vi "Is Connected.vi"(8 "error in (no error)":errorcluster, 9 "Raise error if not connected":bool, 11 "WAMP Client in":refnum<class "WAMP Client.lvclass">) -> (0 "error out":errorcluster, 1 "Is Connected?":bool, 3 "WAMP Client out":refnum<class "WAMP Client.lvclass">)   [LabVIEW 2020, in "wamplv.lvlib" / "WAMP Client.lvclass"]
uses:
  WAMP Client.lvclass
  WAMP Client.lvclass/WAMP Client.ctl
  <vilib>/Utility/error.llb/Error Cluster From Error Code.vi
  <vilib>/ErrorRing/Error Ring.xnode
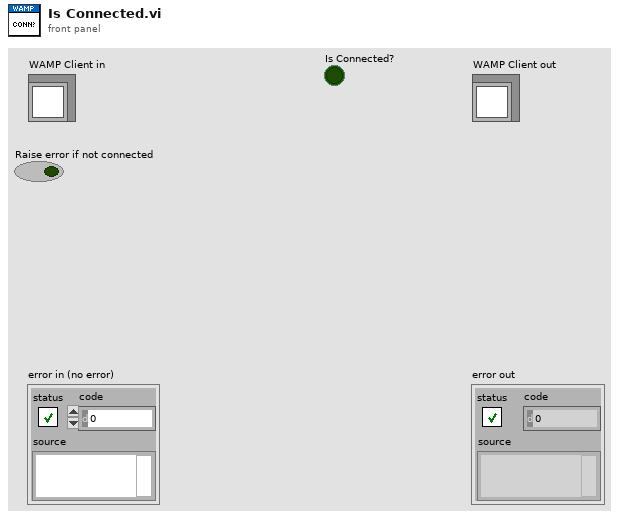
[diagram p1: front panel]
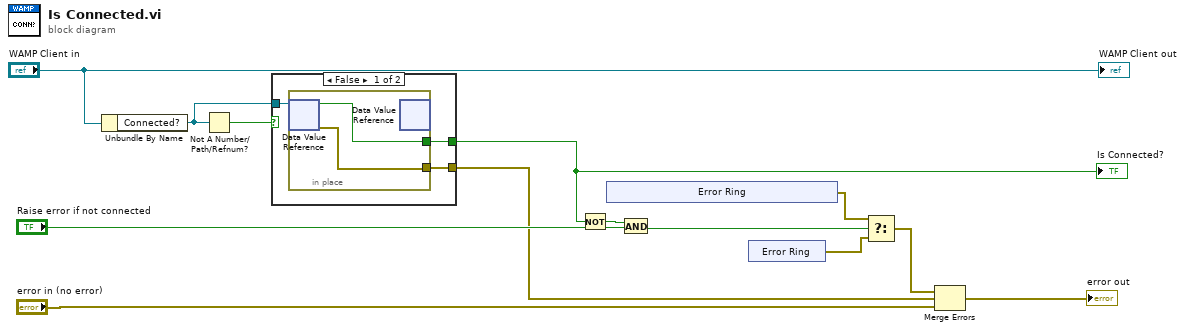
[diagram p0: block diagram]
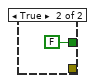
[diagram p2: hidden frame]
diagram:
  n1 = Unbundle By Name("WAMP Client in") -> ("Connected?"=w1:refnum<data-value>)
  n2 = Not A Number/Path/Refnum?(number/path/refnum=w1) -> (NaN/Path/Refnum?=w2:bool)
  n3 = case shown="False" w2 {
    tunnel: [w16 FALSE] -> w12
    tunnel: [w15 _] -> w5
    tunnel: w1 -> [w14 _]
    frame False {
      n4 = in-place {
        in-place-border: [w18] -> w16
        in-place-border: [w17] -> w15
        n5 = in-place-dvr #1(w14) -> (w18:bool, w17:errorcluster)
        n6 = in-place-dvr #1() -> ()  [unwired: 1 in, 2 out]
      }
    }
    frame True {
    }
  }
  "Is Connected?" <- w12
  n7 = Not(x=w12) -> (.not. x?=w11:bool)
  n8 = xnode "Error Ring"() -> ("error out"=w9:errorcluster)
  n9 = And(x=w11, y="Raise error if not connected") -> (x .and. y?=w8:bool)
  n10 = xnode "Error Ring"() -> ("error out"=w7:errorcluster)
  n11 = Select(t=w9, s=w8, f=w7) -> (s? t:f=w4:errorcluster)
  n12 = Merge Errors(w4, w5, "error in (no error)") -> (→"error out":errorcluster)
  "WAMP Client out" <- "WAMP Client in"
